vi "temperatura_PH.vi"() -> ()   [LabVIEW 2021]
uses:
  <vilib>/Analysis/baseanly.llb/Mean (DBL).vi
  <vilib>/Analysis/NI_AALBase.lvlib
panel:
  in  "stop":bool
  out "Temperatura średnia":dbl(slide) scale=0.0..100.0
  in  "Składowa zmienna temperatury":dbl(knob) scale=0.0..10.0
  in  "Składowa stała temperatury":dbl
  out "Wyniki rejestracji temperatury":dbl[](graph)
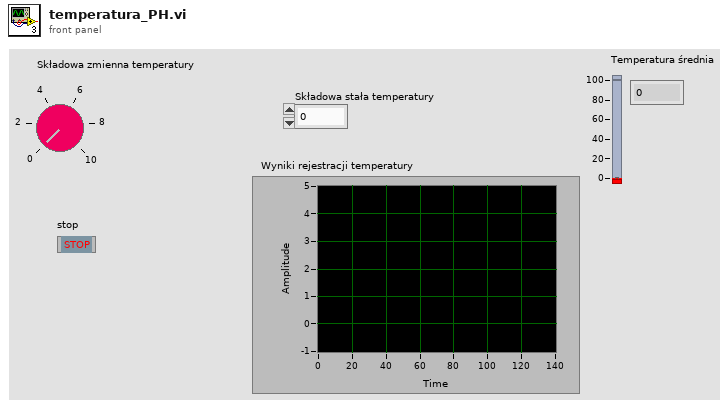
[diagram p1: front panel]
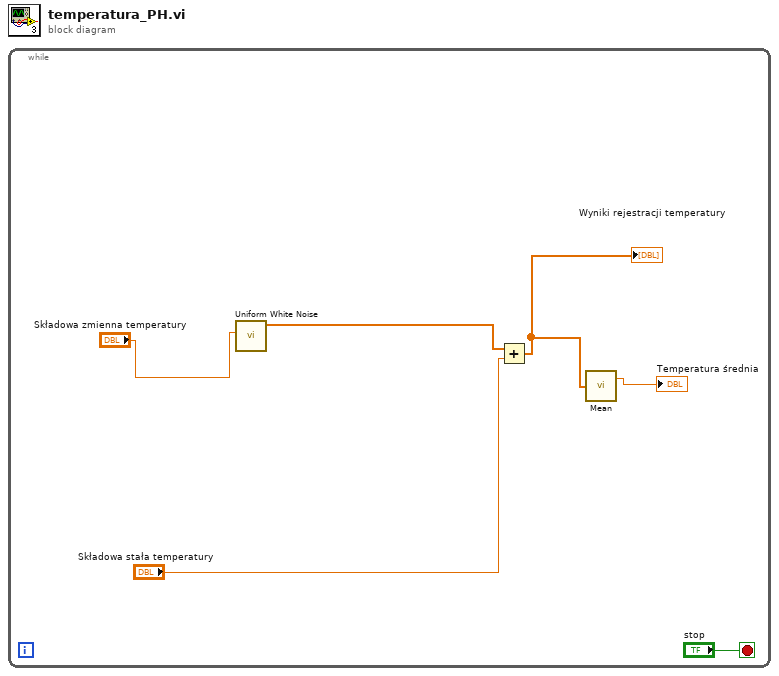
[diagram p0: block diagram]
diagram:
  n1 = while {
    stop <- "stop" stop-if-true
    n2 = call <vilib>:"Uniform White Noise.vi"("amplitude"="Składowa zmienna temperatury") -> ("uniform white noise"=w5:dbl[])  [unwired: 9 in, 1 out]
    n3 = Add(x=w5, y="Składowa stała temperatury") -> (x+y=w4:dbl[])
    "Wyniki rejestracji temperatury" <- w4
    n4 = call-poly <vilib>:"Mean.vi"("X"=w4) -> ("mean"=→"Temperatura średnia":dbl)  [unwired: 1 out]
  }
